vi "Clean up Interface type.vi"(8 "error in (no error)":errorcluster, 11 "VISA Refnum in":refnum<visa-resource-name>) -> (0 "error out":errorcluster, 3 "VISA Refnum out":refnum<visa-resource-name>)   [LabVIEW 2013, in "SetUp VIs.lvlib"]
uses:
  SetUp VIs.lvlib
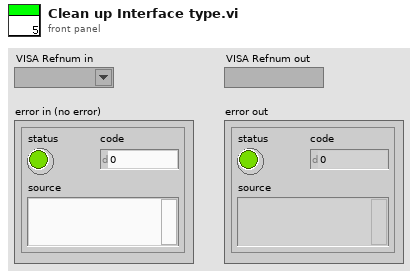
[diagram p1: front panel]
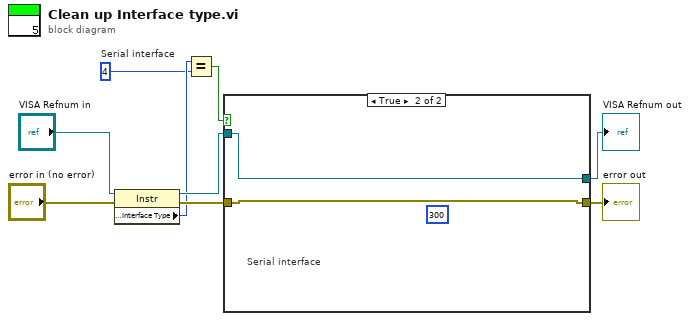
[diagram p0: block diagram]
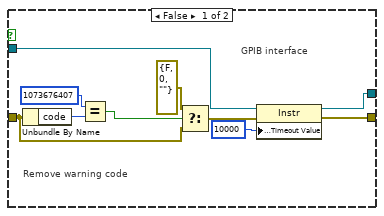
[diagram p2: hidden frame]
diagram:
  w3 = u16 4  # Serial interface
  n1 = property class="Instr"(reference="VISA Refnum in", error in="error in (no error)") -> (reference out=w6:refnum<visa-resource-name>, error out=w7:errorcluster, "Interface Information:Interface Type"=w4:u16)
  n2 = Equal?(x=w4, y=w3) -> (x = y?=w5:bool)
  n3 = case shown="True" w5 {
    tunnel: [w19 w21] -> w8
    tunnel: [w18 w20] -> w9
    tunnel: w6 -> [w17 w21]
    tunnel: w7 -> [w12 w20]
    frame False {
      # "GPIB interface"
      # "Remove warning code"
      n4 = Unbundle By Name(w12) -> ("code"=w15:i32)
      n5 = Equal?(x=1073676407, y=w15) -> (x = y?=w13:bool)
      n6 = Select(t=errorcluster {"status"=FALSE, "code"=0, "source"=""}, s=w13, f=w12) -> (s? t:f=w10:errorcluster)
      n7 = property class="Instr"(reference=w17, error in=w10, "General Settings:Timeout Value"=u32 10000 ("Tmo Value")) -> (reference out=w19:refnum<visa-resource-name>, error out=w18:errorcluster)
    }
    frame True {
      (unwired) u32 300 ("Tmo Value")
      # "Serial interface"
    }
  }
  "error out" <- w9
  "VISA Refnum out" <- w8
